vi "Set ID.vi"(10 "id":i32, 11 "Plugin in":refnum<class "Thread Parameters.lvclass">) -> (3 "Plugin out":refnum<class "Thread Parameters.lvclass">)   [LabVIEW 2017, in "Data Sharing Framework Core.lvlib" / "Data Sharing Framework Engine.lvlib" / "Thread Parameters.lvclass"]
uses:
  Thread Parameters.lvclass
  Thread Parameters.lvclass/Thread Parameters.ctl
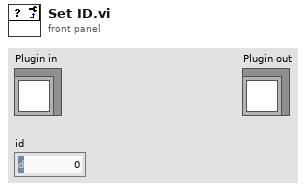
[diagram p1: front panel]
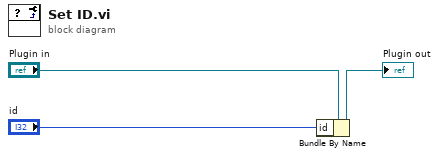
[diagram p0: block diagram]
diagram:
  n1 = Bundle By Name(cluster="Plugin in", "id"="id") -> (→"Plugin out":refnum<class "Thread Parameters.lvclass">)
